vi "FFTtoR,Theta (1D).VI"(0 "X":dbl[](array[numeric]) format="%.2f") -> (1 "+Freq. Mag of FFT":dbl[](array[numeric]) min=0.0 max=127.0 format="%.2f", 2 "+Freq Theta of FFT":dbl[](array[numeric]) min=0.0 max=127.0 format="%.2f")   [LabVIEW 2020]
uses:
  <vilib>/Analysis/2dsp.llb/Real FFT.vi
  <vilib>/Analysis/NI_AALPro.lvlib
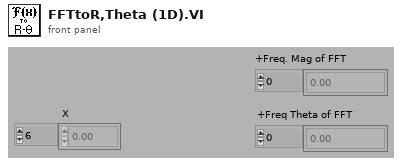
[diagram p1: front panel]
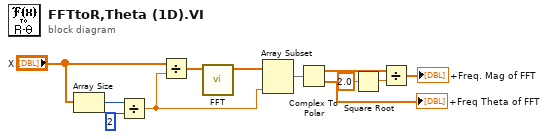
[diagram p0: block diagram]
diagram:
  n1 = Array Size(array="X") -> (size(s)=w11:i32)
  n2 = Divide(x=w11, y=2) -> (x/y=w6:dbl)
  n3 = Divide(x="X", y=w6) -> (x/y=w5:dbl[])
  n4 = call-poly <vilib>:"FFT.vi"("X"=w5) -> ("FFT {X}"=w9:cdb[])  [unwired: 9 in, 1 out]
  n5 = Array Subset(array=w9, length=w6) -> (w8:cdb[])  [unwired: 1 in]
  n6 = Complex To Polar(r * e^(i*theta)=w8) -> (r=w2:dbl[], theta=→"+Freq Theta of FFT":dbl[])
  n7 = Square Root(x=2.0) -> (sqrt(x)=w3:dbl)
  n8 = Divide(x=w2, y=w3) -> (x/y=→"+Freq. Mag of FFT":dbl[])
